vi "Test Method No Arguments.vi"(8 "error in (no error)":errorcluster, 11 "Mock In":refnum<class "Mock.lvclass">) -> (0 "error out":errorcluster, 3 "Mock Out":refnum<class "Mock.lvclass">)   [LabVIEW 2020, in "Mock.lvclass"]
uses:
  Mock.lvclass
  Mock.lvclass/Mock.ctl
  Expectation/Expectation.lvclass
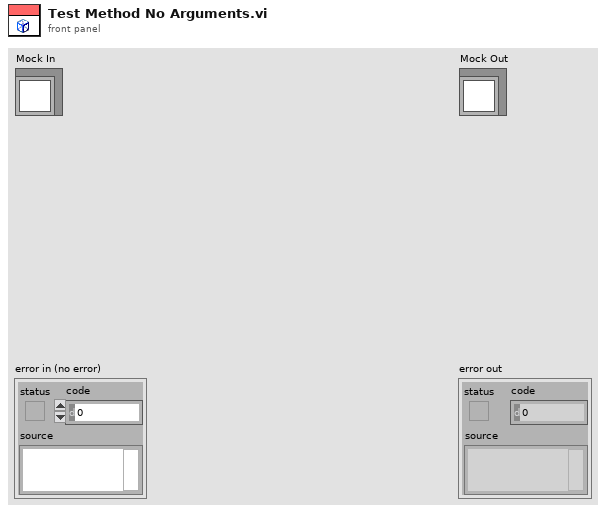
[diagram p1: front panel]
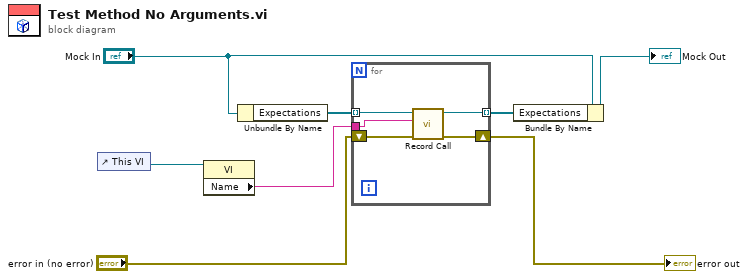
[diagram p0: block diagram]
diagram:
  n1 = control-ref of="This VI"() -> (w8:refnum<vi>)
  n2 = property class="VI"(reference=w8) -> ("Name"=w1:string)  [unwired: 1 in, 2 out]
  n3 = Unbundle By Name("Mock In") -> ("Expectations"=w5:refnum<class "Expectation.lvclass">[])
  n4 = for {
    tunnel: w5 -> [w13] mode=indexing
    tunnel: [w12] -> w4 mode=indexing
    shift-right: [w11] -> w3
    shift-left: "error in (no error)" -> [w10]
    tunnel: w1 -> [w9]
    n5 = call-dynamic "Record Call.vi"("error in (no error)"=w10, "VI Name"=w9, "Expectation in"=w13) -> ("error out"=w11:errorcluster, "Expectation out"=w12:refnum<class "Expectation.lvclass">)  [unwired: 7 in]
  }
  "error out" <- w3
  n6 = Bundle By Name(cluster="Mock In", "Expectations"=w4) -> (→"Mock Out":refnum<class "Mock.lvclass">)
